vi "initiate.vi"(0 "reference in":refnum<class "Subject Controller.lvclass">, 5 "error in (no error)":errorcluster) -> (14 "reference out":refnum<class "Subject Controller.lvclass">, 19 "error out":errorcluster)   [LabVIEW 2015, in "Subject Controller.lvclass"]
uses:
  Subject Controller.lvclass
  File Controller_llb/File Controller.lvclass
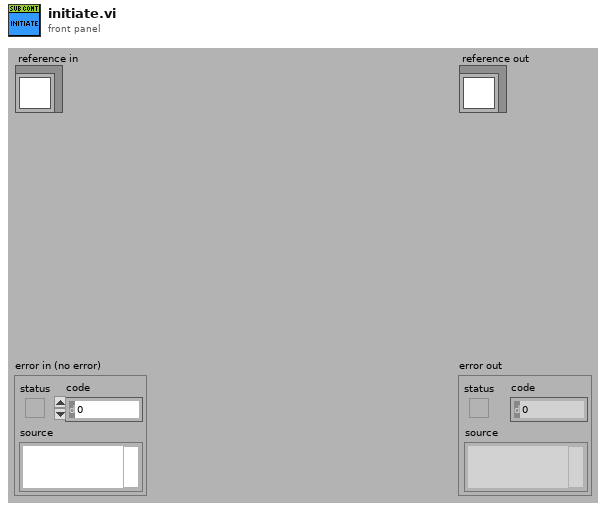
[diagram p1: front panel]
types:
  T1 = typedef "Subject Controller.lvclass/ObjectAttributesRef.ctl" = refnum<data-value>
  T2 = typedef "Subject Controller.lvclass/ObjectAttributes.ctl" = cluster{"MyAttribute":dbl, "subject_controller_ref":refnum<class "Subject Controller.lvclass">, "file_controller_ref":refnum<class "File Controller.lvclass">, "subject_refs":refnum<class "subject.lvclass">[], "subjectIndex":i32, "file_type":T3}
  T3 = typedef "excelFile.lvclass/fileType.ctl" = enum16{"database", "CosmedTest"}
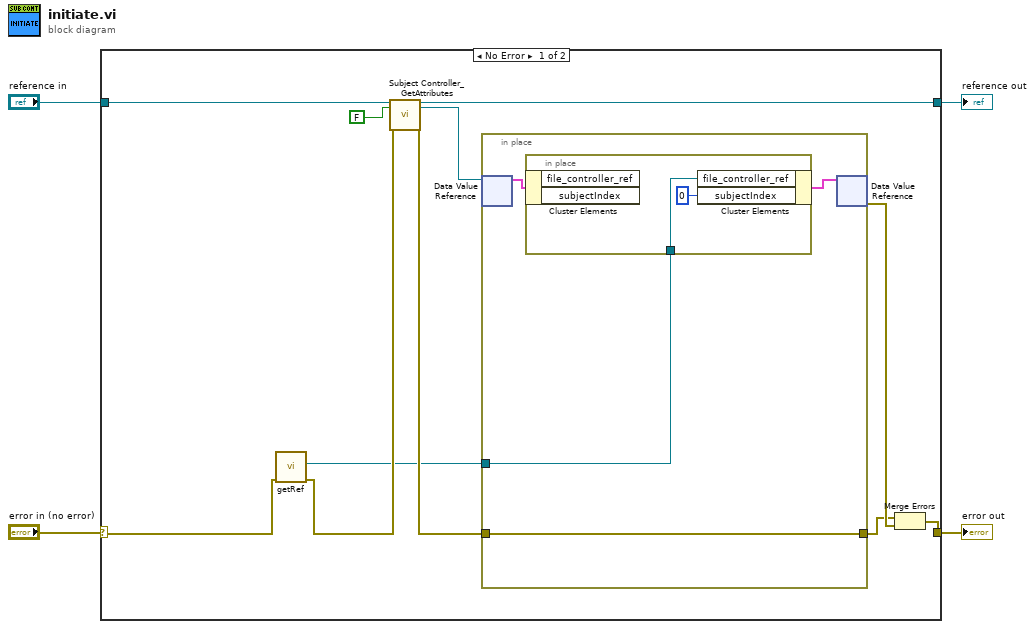
[diagram p0: block diagram]
diagram:
  n1 = case shown="No Error" "error in (no error)" {
    selector: "error in (no error)" -> [w7 w23]
    tunnel: [w15 w23] -> w3
    tunnel: [w9 w22] -> w1
    tunnel: "reference in" -> [w12 w22]
    frame No Error {
      n2 = call "getRef.vi"("error in (no error)"=w7) -> ("error out"=w6:errorcluster, "File Controller.lvclass"=w5:refnum<class "File Controller.lvclass">)  [unwired: 9 in]
      n3 = call "Subject Controller_GetAttributes.vi"("reference in"=w12, "return data? (T)"=FALSE, "error in (no error)"=w6) -> ("reference out"=w9:refnum<class "Subject Controller.lvclass">, "attributes ref"=w8:T1, "error out"=w10:errorcluster)  [unwired: 13 in, 1 out]
      n4 = in-place {
        in-place-border: w10 -> [w17]
        in-place-border: [w17] -> w13
        in-place-border: w5 -> [w16]
        n5 = in-place-dvr #1(w8) -> (w18:T2)  [unwired: 1 out]
        n6 = in-place {
          in-place-border: w16 -> [w21]
          n7 = in-place-cluster #2(w18) -> ()  [unwired: 2 out]
          n8 = in-place-cluster #2("file_controller_ref"=w21, "subjectIndex"=0) -> (w19:T2)
        }
        n9 = in-place-dvr #1(w19) -> (w14:errorcluster)  [unwired: 1 out]
      }
      n10 = Merge Errors(w13, w14) -> (w15:errorcluster)
    }
    frame Error {
    }
  }
  "error out" <- w3
  "reference out" <- w1
